vi "Take Step.vi"(8 "error in (no error)":errorcluster, 10 "Maze In":refnum<class "Maze.lvclass">, 11 "Mouse in":refnum<class "Mouse.lvclass">) -> (0 "error out":errorcluster, 2 "Maze":refnum<class "Maze.lvclass">, 3 "Mouse out":refnum<class "Mouse.lvclass">, 5 "Move?":bool, 7 "Bad Action?":bool)   [LabVIEW 2020, in "Maze.lvlib" / "Mouse.lvclass"]
doc: "Takes a step for the mouse instance. Calls the child implementation's Decide Action and then updates the state to reflect that choice. Checks for wall crashes to ensure implementations are monitoring distances properly."
uses:
  Mouse.lvclass
  Maze/Maze.lvclass
  Mouse.lvclass/Mouse.ctl
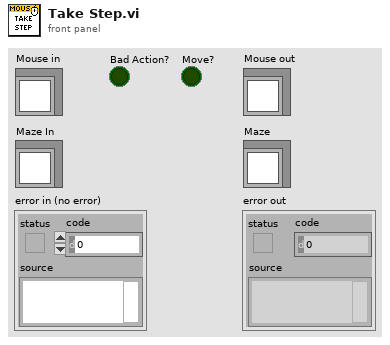
[diagram p1: front panel]
types:
  T1 = typedef "Maze.lvlib/Action.ctl" = enum16{"Turn Left", "Turn Right", "Forward", "*Drop Marker", "*Pickup Marker"}
  T2 = typedef "Maze.lvlib/Direction.ctl" = enum8{"East", "North", "West", "South"}
  T3 = typedef "Maze.lvlib/Position.ctl" = cluster{"S":i32, "E":i32}
  T4 = typedef "Maze.lvlib/Adjacency.ctl" = cluster{"E":bool, "N":bool, "W":bool, "S":bool, "Goal":bool, "Start":bool}
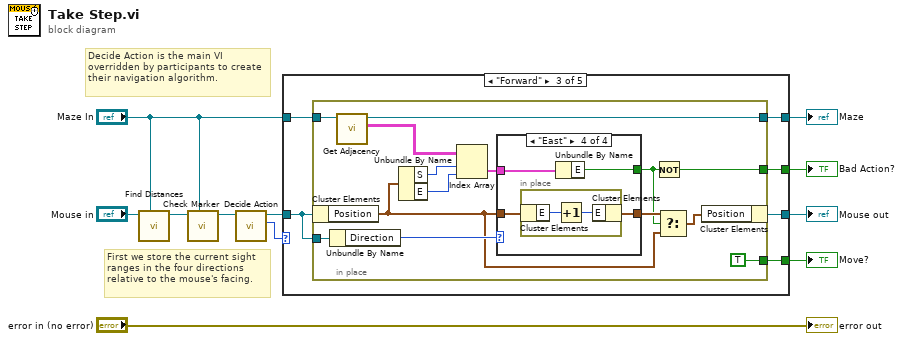
[diagram p0: block diagram]
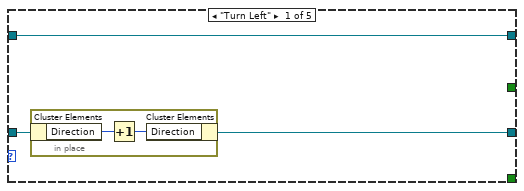
[diagram p2: hidden frame]
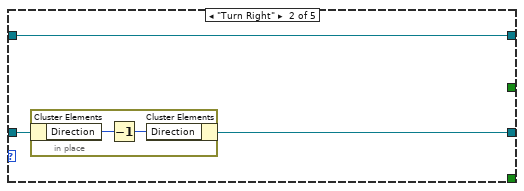
[diagram p3: hidden frame]
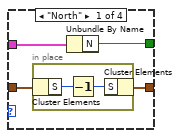
[diagram p4: hidden frame]
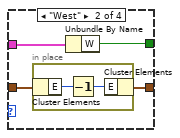
[diagram p5: hidden frame]
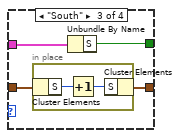
[diagram p6: hidden frame]
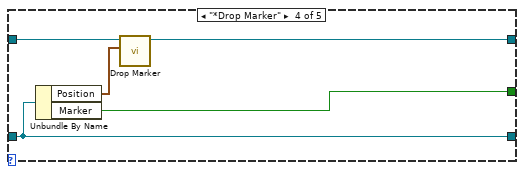
[diagram p7: hidden frame]
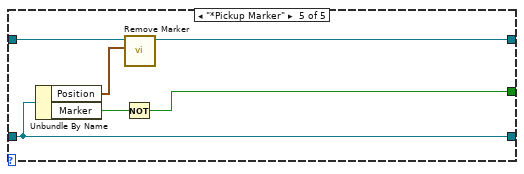
[diagram p8: hidden frame]
diagram:
  # "Decide Action is the main VI overridden by participants to create their navigation algorithm."
  # "First we store the current sight ranges in the four directions relative to the mouse's facing."
  n1 = call "Find Distances.vi"("Maze"="Maze In", "Mouse in"="Mouse in") -> ("Mouse out"=w5:refnum<class "Mouse.lvclass">)  [unwired: 9 in]
  n2 = call "Check Marker.vi"("Maze"="Maze In", "Mouse in"=w5) -> ("Mouse out"=w4:refnum<class "Mouse.lvclass">)  [unwired: 8 in, 1 out]
  n3 = call-dynamic "Decide Action.vi"("Mouse in"=w4) -> ("Action"=w10:T1, "Mouse out"=w9:refnum<class "Mouse.lvclass">)  [unwired: 8 in, 1 out]
  n4 = case shown="\"Forward\"" w10 {
    tunnel: w9 -> [w14 w19 w27 w66 w75]
    tunnel: [w13 w18 w24 w66 w75] -> w6
    tunnel: "Maze In" -> [w12 w17 w26 w70 w74]
    tunnel: [_ _ w25 w68 w71] -> w8
    tunnel: [_ _ w23 _ _] -> w7
    tunnel: [w12 w17 w22 w67 w72] -> w1
    frame "Turn Left" {
      n5 = in-place {
        n6 = in-place-cluster #1(w14) -> ("Direction"=w16:T2)
        n7 = Increment(x=w16) -> (x+1=w15:T2)
        n8 = in-place-cluster #1("Direction"=w15) -> (w13:refnum<class "Mouse.lvclass">)
      }
    }
    frame "Turn Right" {
      n9 = in-place {
        n10 = in-place-cluster #2(w19) -> ("Direction"=w21:T2)
        n11 = Decrement(x=w21) -> (x-1=w20:T2)
        n12 = in-place-cluster #2("Direction"=w20) -> (w18:refnum<class "Mouse.lvclass">)
      }
    }
    frame "Forward" {
      n13 = in-place {
        in-place-border: w27 -> [w41]
        in-place-border: w26 -> [w40]
        in-place-border: [w30] -> w25
        in-place-border: [TRUE] -> w23
        in-place-border: [w28] -> w22
        n14 = in-place-cluster #3(w27) -> ("Position"=w33:T3)
        n15 = Unbundle By Name(w41) -> ("Direction"=w35:T2)
        n16 = call "Get Adjacency.vi"("Maze in"=w40) -> ("Adjacency"=w39:T4[][], "Maze out"=w28:refnum<class "Maze.lvclass">)  [unwired: 8 in, 1 out]
        n17 = Unbundle By Name(w33) -> ("S"=w37:i32, "E"=w38:i32)
        n18 = Index Array(array=w39, index (row)=w37, index (col)=w38) -> (element=w36:T4)
        n19 = case shown="\"East\"" w35 {
          tunnel: w36 -> [w43 w49 w55 w61]
          tunnel: w33 -> [w45 w51 w57 w63]
          tunnel: [w44 w50 w56 w62] -> w34
          tunnel: [w42 w48 w54 w60] -> w31
          frame "North" {
            n20 = in-place {
              n21 = in-place-cluster #4(w45) -> ("S"=w47:i32)
              n22 = Decrement(x=w47) -> (x-1=w46:i32)
              n23 = in-place-cluster #4("S"=w46) -> (w44:T3)
            }
            n24 = Unbundle By Name(w43) -> ("N"=w42:bool)
          }
          frame "West" {
            n25 = in-place {
              n26 = in-place-cluster #5(w51) -> ("E"=w53:i32)
              n27 = Decrement(x=w53) -> (x-1=w52:i32)
              n28 = in-place-cluster #5("E"=w52) -> (w50:T3)
            }
            n29 = Unbundle By Name(w49) -> ("W"=w48:bool)
          }
          frame "South" {
            n30 = in-place {
              n31 = in-place-cluster #6(w57) -> ("S"=w59:i32)
              n32 = Increment(x=w59) -> (x+1=w58:i32)
              n33 = in-place-cluster #6("S"=w58) -> (w56:T3)
            }
            n34 = Unbundle By Name(w55) -> ("S"=w54:bool)
          }
          frame "East" {
            n35 = in-place {
              n36 = in-place-cluster #7(w63) -> ("E"=w65:i32)
              n37 = Increment(x=w65) -> (x+1=w64:i32)
              n38 = in-place-cluster #7("E"=w64) -> (w62:T3)
            }
            n39 = Unbundle By Name(w61) -> ("E"=w60:bool)
          }
        }
        n40 = Not(x=w31) -> (.not. x?=w30:bool)
        n41 = Select(t=w34, s=w31, f=w33) -> (s? t:f=w32:T3)
        n42 = in-place-cluster #3("Position"=w32) -> (w24:refnum<class "Mouse.lvclass">)
      }
    }
    frame "*Drop Marker" {
      n43 = Unbundle By Name(w66) -> ("Position"=w69:T3, "Marker"=w68:bool)
      n44 = call "Drop Marker.vi"("Position"=w69, "Maze in"=w70) -> ("Maze out"=w67:refnum<class "Maze.lvclass">)  [unwired: 8 in, 1 out]
    }
    frame "*Pickup Marker" {
      n45 = Unbundle By Name(w75) -> ("Position"=w73:T3, "Marker"=w76:bool)
      n46 = Not(x=w76) -> (.not. x?=w71:bool)
      n47 = call "Remove Marker.vi"("Position"=w73, "Maze in"=w74) -> ("Maze out"=w72:refnum<class "Maze.lvclass">)  [unwired: 8 in, 1 out]
    }
  }
  "Mouse out" <- w6
  "Bad Action?" <- w8
  "Move?" <- w7
  "Maze" <- w1
  "error out" <- "error in (no error)"
